vi "Close.vi"(8 "error in (no error)":errorcluster, 10 "skvc in":string[][](array[string]), 11 "Ini Path in":path) -> (0 "error out":errorcluster, 3 "Ini Path out":path)   [LabVIEW 2021, in "Config.lvlib"]
uses:
  Config.lvlib
  <vilib>/Utility/error.llb/Error Cluster From Error Code.vi
  <vilib>/ErrorRing/Error Ring.xnode
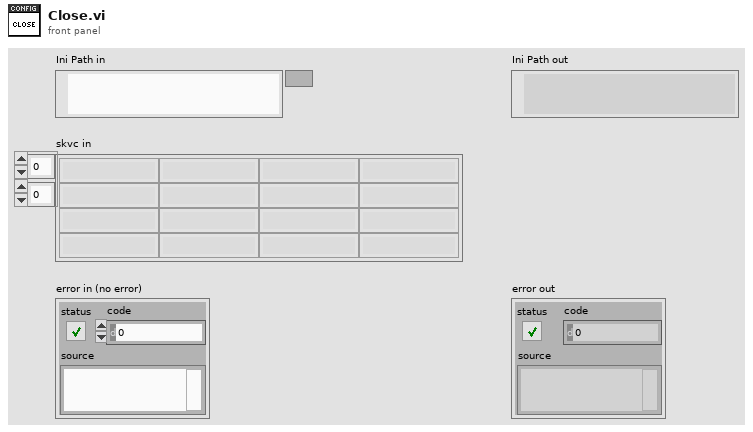
[diagram p1: front panel]
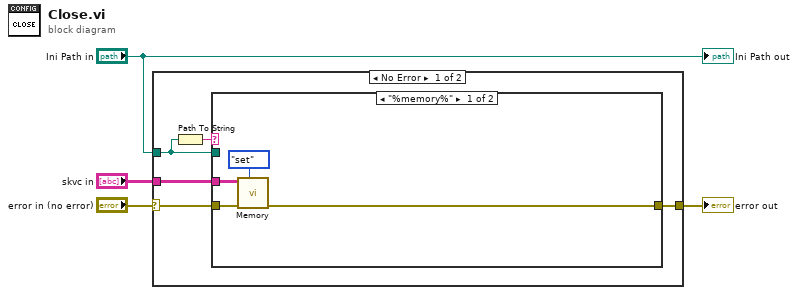
[diagram p0: block diagram]
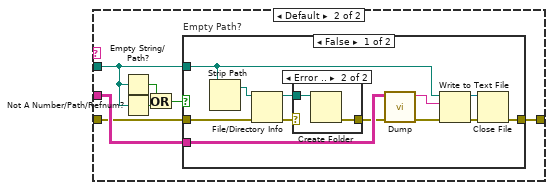
[diagram p2: hidden frame]
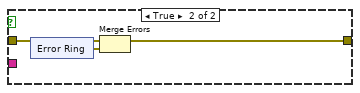
[diagram p4: hidden frame]
diagram:
  n1 = case shown="No Error" "error in (no error)" {
    selector: "error in (no error)" -> [w8 w43]
    tunnel: [w9 w43] -> w4
    tunnel: "Ini Path in" -> [w6 _]
    tunnel: "skvc in" -> [w5 _]
    frame No Error {
      n2 = Path To String(path=w6) -> (string=w7:string)
      n3 = case shown="\"%memory%\"" w7 {
        tunnel: [w12 w18] -> w9
        tunnel: w8 -> [w11 w16]
        tunnel: w6 -> [_ w15]
        tunnel: w5 -> [w10 w17]
        frame "%memory%" {
          n4 = call "Memory.vi"("Action (get)"=enum8{"get", "set"}."set", "error in (no error)"=w11, "skvc in"=w10) -> ("error out"=w12:errorcluster)  [unwired: 7 in, 1 out]
        }
        frame Default {
          n5 = Empty String/Path?(string/path=w15) -> (empty?=w19:bool)
          n6 = Not A Number/Path/Refnum?(number/path/refnum=w15) -> (NaN/Path/Refnum?=w20:bool)
          n7 = Or(x=w19, y=w20) -> (x .or. y?=w14:bool)
          n8 = case "Empty Path?" shown="False" w14 {
            tunnel: [w21 w36] -> w18
            tunnel: w17 -> [w29 _]
            tunnel: w16 -> [w24 w37]
            tunnel: w15 -> [w22 _]
            frame False {
              n9 = Strip Path(path=w22) -> (stripped path=w26:path)  [unwired: 1 out]
              n10 = File/Directory Info(path=w26, error in=w24) -> (path out=w25:path, error out=w27:errorcluster)  [unwired: 5 out]
              n11 = case shown="Error .." w27 {
                selector: w27 -> [w33 _]
                tunnel: [w33 w35] -> w23
                tunnel: w25 -> [_ w34]
                frame No Error {
                }
                frame Error {
                  n12 = Create Folder(path (use dialog)=w34) -> (error out=w35:errorcluster)  [unwired: 2 in, 2 out]
                }
              }
              n13 = call "Dump.vi"("error in (no error)"=w23, "skvc"=w29) -> ("error out"=w30:errorcluster, "Text"=w28:string)  [unwired: 8 in]
              n14 = Write to Text File(file (use dialog)=w22, text=w28, error in=w30) -> (refnum out=w31:refnum<file>, error out=w32:errorcluster)  [unwired: 1 in, 1 out]
              n15 = Close File(refnum=w31, error in=w32) -> (error out=w21:errorcluster)  [unwired: 1 out]
            }
            frame True {
              n16 = xnode "Error Ring"() -> ("error out"=w38:errorcluster)
              n17 = Merge Errors(w37, w38) -> (w36:errorcluster)
            }
          }
        }
      }
    }
    frame Error {
    }
  }
  "error out" <- w4
  "Ini Path out" <- "Ini Path in"
